vi "SpecAn Fetch ACP.vi"(0 "RFmx Handle In":refnum<k21>, 1 "Selector String":string, 11 "error in (no error)":errorcluster) -> (4 "RFmx Handle Out":refnum<k21>, 6 "ACP Results":T1 {"Total Carrier Power (dBm or dBm/Hz)" format="%.2f"}, 15 "error out":errorcluster)   [LabVIEW 2016, in "RFmxSpecAn.lvlib"]
uses:
  RFmxSpecAn.lvlib
  Typedefs/SpecAn ACP Results.ctl
  Typedefs/SpecAn ACP Offset Results.ctl
  Typedefs/SpecAn ACP Component Carrier Results.ctl
  <vilib>/RFmx/SpecAn/mx/RFmxSpecAn.llb/RFmxSpecAn Build Signal String.vi
  <vilib>/RFmx/RFInstr/mx/RFmxInstr.llb/RFmxInstr Build Signal String.vi
  <vilib>/RFmx/SpecAn/mx/RFmxSpecAn.llb/RFmxSpecAn ACP Fetch Offset Measurement (Array).vi
  <vilib>/RFmx/SpecAn/mx/RFmxSpecAn.llb/RFmxSpecAn ACP Fetch Carrier Measurement.vi
  <vilib>/RFmx/SpecAn/mx/RFmxSpecAn.llb/RFmxSpecAn ACP Fetch Total Carrier Power.vi
  <resource>/objmgr/RFmxSpecAn.rc
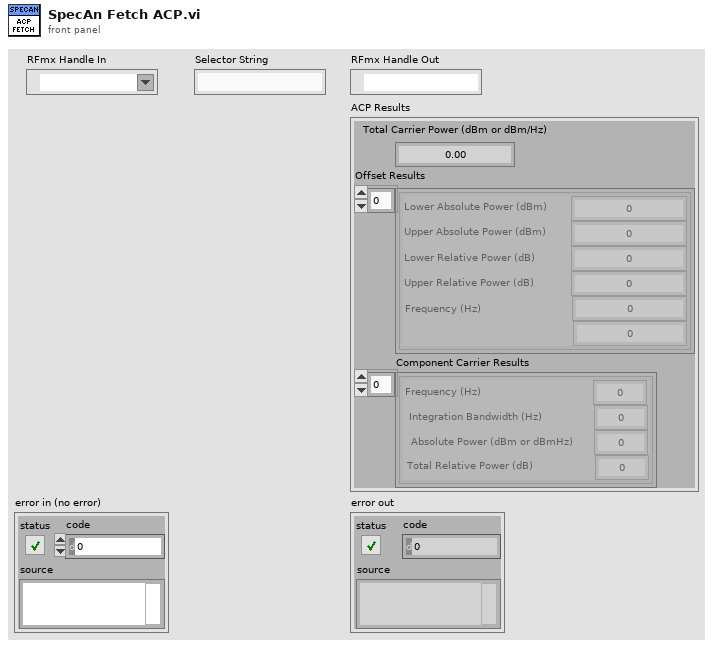
[diagram p1: front panel]
types:
  T1 = typedef "RFmxSpecAn.lvlib/SpecAn ACP Results.ctl" = cluster{"Total Carrier Power (dBm or dBm/Hz)":dbl, "Offset Results":T2[], "Component Carrier Results":T3[]}
  T2 = typedef "RFmxSpecAn.lvlib/SpecAn ACP Offset Results.ctl" = cluster{"Lower Absolute Power (dBm)":dbl, "Upper Absolute Power (dBm)":dbl, "Lower Relative Power (dB)":dbl, "Upper Relative Power (dB)":dbl, "Frequency (Hz)":dbl, "Integration Bandwidth (Hz)":dbl}
  T3 = typedef "RFmxSpecAn.lvlib/SpecAn ACP Component Carrier Results.ctl" = cluster{"Frequency (Hz)":dbl, "Integration Bandwidth (Hz)":dbl, "Absolute Power (dBm or dBmHz)":dbl, "Total Relative Power (dB)":dbl}
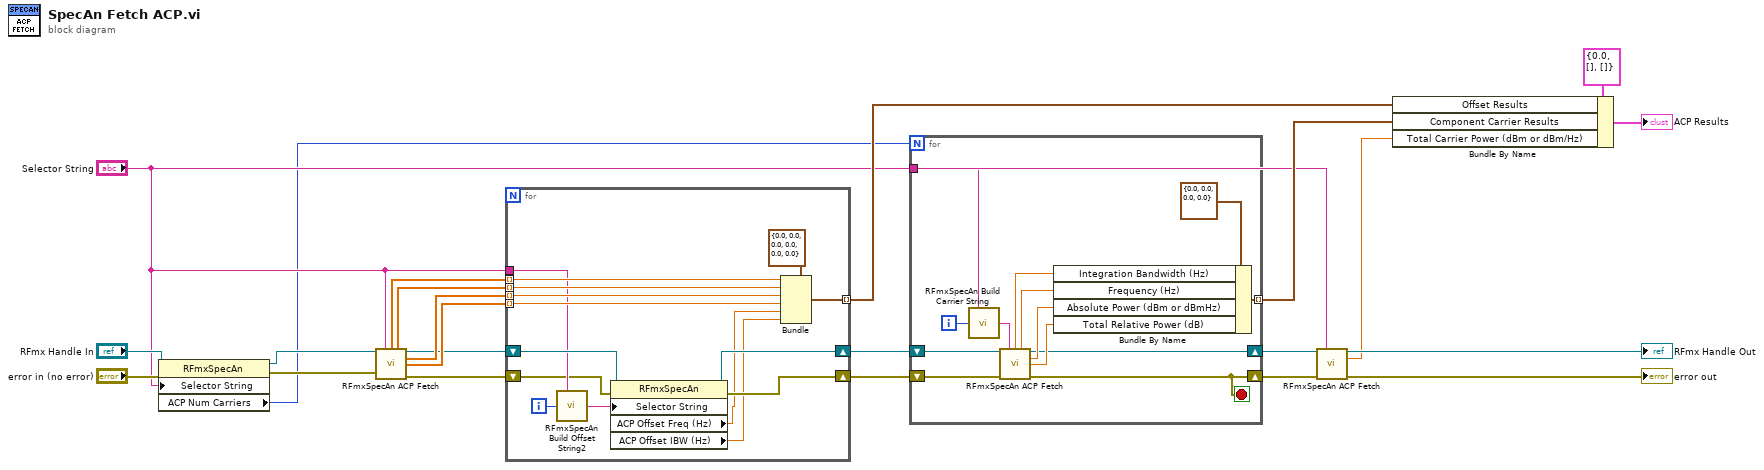
[diagram p0: block diagram]
diagram:
  n1 = property class="RFmxSpecAn"(reference="RFmx Handle In", error in="error in (no error)", "Selector String"="Selector String") -> (reference out=w3:refnum<k21>, error out=w5:errorcluster, "ACP Num Carriers"=w1:i32)
  n2 = call-poly <vilib>:"RFmxSpecAn ACP Fetch.vi"("Instrument Handle In"=w3, "Selector String"="Selector String", "error in (no error)"=w5) -> ("Lower Absolute Power (dBm or dBm/Hz)"=w19:dbl[], "Upper Absolute Power (dBm or dBm/Hz)"=w18:dbl[], "Instrument Handle Out"=w14:refnum<k21>, "Lower Relative Power (dB)"=w17:dbl[], "Upper Relative Power (dB)"=w16:dbl[], "error out"=w15:errorcluster)  [unwired: 7 in]
  n3 = for {
    shift-right: [w37] -> w10
    shift-left: w14 -> [w35]
    shift-right: [w38] -> w9
    shift-left: w15 -> [w24]
    tunnel: [w36] -> w11 mode=indexing
    tunnel: w19 -> [w34] mode=indexing
    tunnel: w18 -> [w33] mode=indexing
    tunnel: w17 -> [w32] mode=indexing
    tunnel: w16 -> [w31] mode=indexing
    tunnel: "Selector String" -> [w29]
    i -> [w28]
    n4 = call <vilib>:"RFmxSpecAn Build Offset String2.vi"("Selector String"=w29, "Offset Number"=w28) -> ("Selector String Out"=w25:string)  [unwired: 13 in]
    n5 = property class="RFmxSpecAn"(reference=w35, error in=w24, "Selector String"=w25) -> (reference out=w37:refnum<k21>, error out=w38:errorcluster, "ACP Offset Freq (Hz)"=w26:dbl, "ACP Offset IBW (Hz)"=w27:dbl)
    n6 = Bundle(cluster=T2 {"Lower Absolute Power (dBm)"=0.0, "Upper Absolute Power (dBm)"=0.0, "Lower Relative Power (dB)"=0.0, "Upper Relative Power (dB)"=0.0, "Frequency (Hz)"=0.0, "Integration Bandwidth (Hz)"=0.0} ("ACP Offset Results"), "Lower Absolute Power (dBm)"=w34, "Upper Absolute Power (dBm)"=w33, "Lower Relative Power (dB)"=w32, "Upper Relative Power (dB)"=w31, "Frequency (Hz)"=w26, "Integration Bandwidth (Hz)"=w27) -> (w36:T2)
  }
  n7 = for {
    N: w1 -> [_]
    shift-right: [w45] -> w23
    shift-left: w10 -> [w51]
    shift-right: [w43] -> w22
    shift-left: w9 -> [w50]
    tunnel: [w46] -> w8 mode=indexing
    tunnel: "Selector String" -> [w41]
    i -> [w40]
    stop <- w43 stop-if-true
    n8 = call <vilib>:"RFmxSpecAn Build Carrier String.vi"("Signal Name"=w41, "Carrier Number"=w40) -> ("Carrier String"=w42:string)  [unwired: 13 in]
    n9 = call-poly <vilib>:"RFmxSpecAn ACP Fetch.vi"("Instrument Handle In"=w51, "Selector String"=w42, "error in (no error)"=w50) -> ("Integration Bandwidth (Hz)"=w44:dbl, "Frequency (Hz)"=w49:dbl, "Instrument Handle Out"=w45:refnum<k21>, "Absolute Power (dBm or dBm/Hz)"=w48:dbl, "Total Relative Power (dB)"=w47:dbl, "error out"=w43:errorcluster)  [unwired: 7 in]
    n10 = Bundle By Name(cluster=T3 {"Frequency (Hz)"=0.0, "Integration Bandwidth (Hz)"=0.0, "Absolute Power (dBm or dBmHz)"=0.0, "Total Relative Power (dB)"=0.0} ("ACP Component Carrier Results"), "Integration Bandwidth (Hz)"=w44, "Frequency (Hz)"=w49, "Absolute Power (dBm or dBmHz)"=w48, "Total Relative Power (dB)"=w47) -> (w46:T3)
  }
  n11 = call-poly <vilib>:"RFmxSpecAn ACP Fetch.vi"("Instrument Handle In"=w23, "Selector String"="Selector String", "error in (no error)"=w22) -> ("Instrument Handle Out"=→"RFmx Handle Out":refnum<k21>, "Total Carrier Power (dBm or dBm/Hz)"=w7:dbl, "error out"=→"error out":errorcluster)  [unwired: 10 in]
  n12 = Bundle By Name(cluster=T1 {"Total Carrier Power (dBm or dBm/Hz)"=0.0, "Offset Results"=[], "Component Carrier Results"=[]} ("ACP Results"), "Offset Results"=w11, "Component Carrier Results"=w8, "Total Carrier Power (dBm or dBm/Hz)"=w7) -> (→"ACP Results":T1)
